vi "ces.vi"() -> ()   [LabVIEW 2014]
panel:
  out "十进制整型字符串":string
  in  "数值":dbl
  out "字符串 2":string="假"
  in  "字符串":string
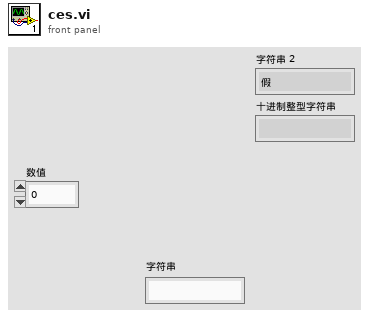
[diagram p1: front panel]
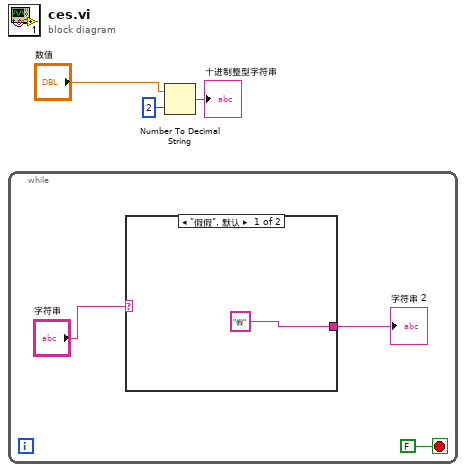
[diagram p0: block diagram]
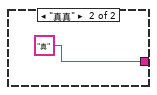
[diagram p2: hidden frame]
diagram:
  n1 = while {
    stop <- FALSE stop-if-true
    n2 = case shown="\"假假\", 默认" "字符串" {
      tunnel: ["假" "真"] -> w4
      frame "假假", Default {
      }
      frame "真真" {
      }
    }
    "字符串 2" <- w4
  }
  n3 = Number To Decimal String(number="数值", width (-)=i16 2 ("宽度(-)")) -> (decimal integer string=→"十进制整型字符串":string)
